vi "LVClass_ClosedLoopSmoothing_Compute_GainFactor.vi"(0 "ClosedLoopSmoothing in":refnum<class "ClosedLoopSmoothing.lvclass">, 5 "gain_factor":sgl, 7 "amplitude":i32, 11 "error in (no error)":errorcluster) -> (4 "ClosedLoopSmoothing out":refnum<class "ClosedLoopSmoothing.lvclass">, 6 "gain_factor":sgl, 15 "error out":errorcluster)   [LabVIEW 2020, in "ClosedLoopSmoothing.lvclass"]
uses:
  ClosedLoopSmoothing.lvclass
  ClosedLoopSmoothing.lvclass/ClosedLoopSmoothing.ctl
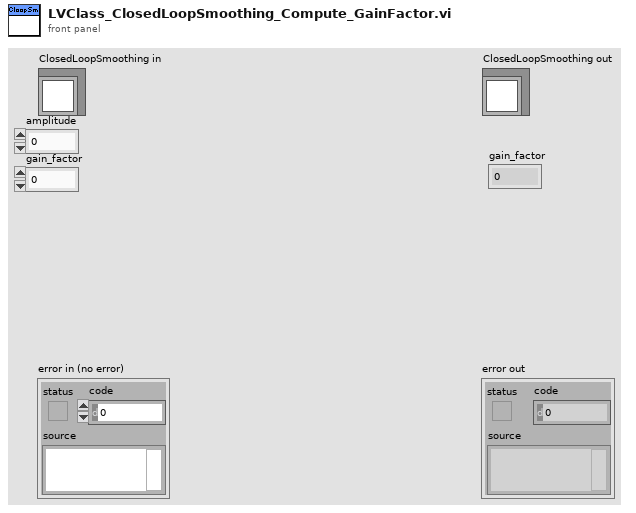
[diagram p1: front panel]
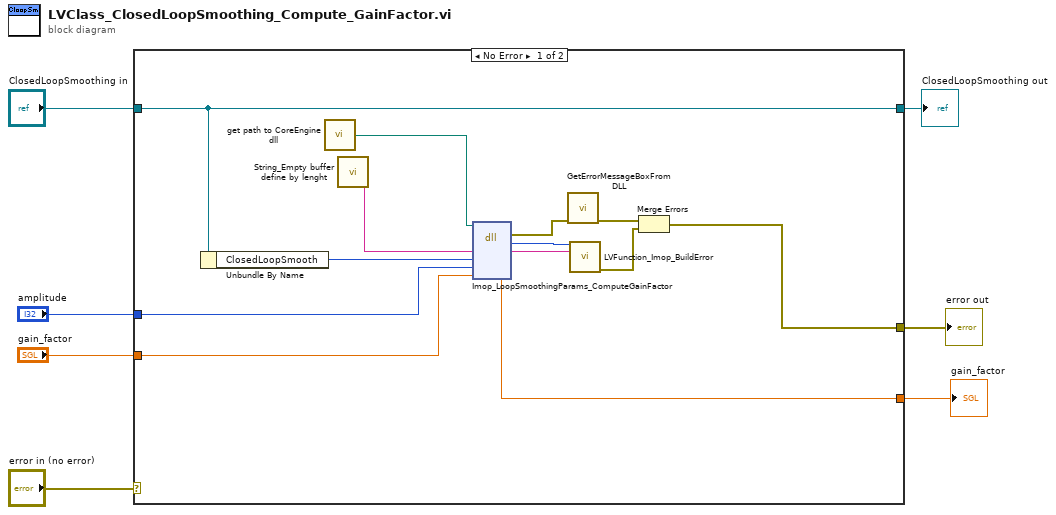
[diagram p0: block diagram]
diagram:
  n1 = case shown="No Error" "error in (no error)" {
    selector: "error in (no error)" -> [_ w22]
    tunnel: [w13 w22] -> w6
    tunnel: [w11 w21] -> w4
    tunnel: "ClosedLoopSmoothing in" -> [w11 w21]
    tunnel: [w8 _] -> w3
    tunnel: "amplitude" -> [w10 _]
    tunnel: "gain_factor" -> [w9 _]
    frame No Error {
      n2 = Unbundle By Name(w11) -> ("ClosedLoopSmooth"=w12:i32)
      n3 = call "get path to CoreEngine dll.vi"() -> ("path to c_interface_vc100.dll"=w14:path)  [unwired: 12 in, 3 out]
      n4 = call "String_Empty buffer define by lenght.vi"() -> ("Empty buffer"=w20:string)  [unwired: 1 in]
      n5 = dll-call lib="D:/soft/HASO_v3/SVN_trunk/ImOpCoreEngine4_LV2011/DLLs/c_interface_vc100.dll" fn="Imop_LoopSmoothingParams_ComputeGainFactor"(path in=w14, "message"=w20, "smoothing_params"=w12, "amplitude"=w10, "gain_factor"=w9) -> (error out=w17:errorcluster, "return type"=w18:i32, "message"=w19:string, "gain_factor"=w8:sgl)  [unwired: 4 in, 1 out]
      n6 = call "GetErrorMessageBoxFromDLL.vi"("error IN"=w17) -> ("error OUT"=w16:errorcluster)  [unwired: 10 in]
      n7 = call "LVFunction_Imop_BuildError.vi"("code"=w18, "String to Prepend to source (\"\")"=w19) -> ("error out"=w15:errorcluster)  [unwired: 13 in]
      n8 = Merge Errors(w16, w15) -> (w13:errorcluster)
    }
    frame Error {
    }
  }
  "error out" <- w6
  "ClosedLoopSmoothing out" <- w4
  "gain_factor" <- w3
